vi "FixAbsolute.vi"(10 "Relative":string) -> (2 "Absolute":string)   [LabVIEW 2020]
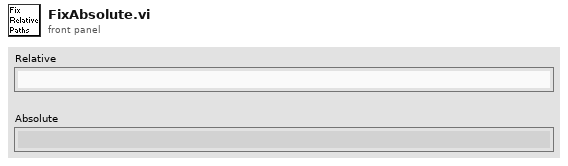
[diagram p1: front panel]
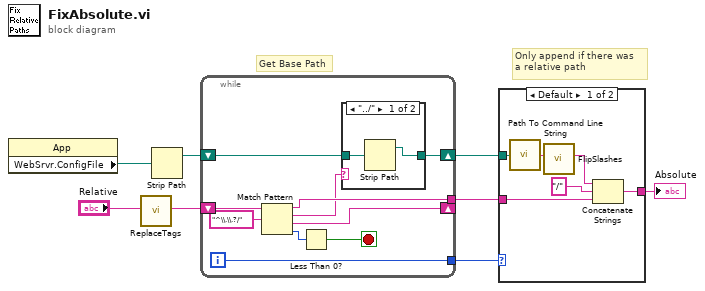
[diagram p0: block diagram]
diagram:
  # "Only append if there was\na relative path"
  # "Get Base Path"
  n1 = property class="App"() -> ("WebSrvr.ConfigFile"=w3:path)  [unwired: 2 in, 2 out]
  n2 = call <vilib>:"ReplaceTags.vi"("Path in"="Relative") -> ("Path out"=w4:string)  [unwired: 10 out]
  n3 = Strip Path(path=w3) -> (stripped path=w2:path)  [unwired: 1 out]
  n4 = while {
    shift-right: [w15] -> _
    shift-left: w4 -> [w18]
    shift-right: [w12] -> w8
    shift-left: w2 -> [w14]
    tunnel: [w11] -> w6
    tunnel: [w9] -> w1
    i -> [w9]
    stop <- w13 stop-if-true
    n5 = Match Pattern(string=w18, regular expression="^\\.\\.?/") -> (before substring=w11:string, match substring=w10:string, after substring=w15:string, offset past match=w16:i32)  [unwired: 1 out]
    n6 = Less Than 0?(x=w16) -> (x < 0?=w13:bool)
    n7 = case shown="\"../\"" w10 {
      tunnel: w14 -> [w20 w21]
      tunnel: [w19 w21] -> w12
      frame "../" {
        n8 = Strip Path(path=w20) -> (stripped path=w19:path)  [unwired: 1 out]
      }
      frame Default {
      }
    }
  }
  n9 = case shown="Default" w1 {
    tunnel: w8 -> [w27 _]
    tunnel: [w25 w28] -> w7
    tunnel: w6 -> [w23 w28]
    frame Default {
      n10 = call <vilib>:"Path To Command Line String.vi"("path"=w27) -> ("string"=w26:string)
      n11 = call <vilib>:"FlipSlashes.vi"("Before"=w26) -> ("After"=w22:string)  [unwired: 1 in, 9 out]
      n12 = Concatenate Strings(w22, "/" ("string"), w23) -> (w25:string)
    }
    frame 0 {
    }
  }
  "Absolute" <- w7
